vi "MyArray_client.vi"() -> ()   [LabVIEW 2010]
uses:
  src/i3-json-1.0.0-10/JSON Generation/Create Value Files/Create Value - Object.vi
  src/i3-json-1.0.0-10/JSON Generation/Add Object Parameter Files/Add Object Parameter - Numeric.vi
  src/i3-json-1.0.0-10/JSON Parsing/Get Array Value at Index Files/Get Array Value at Index - Numeric.vi
  src/i3-json-1.0.0-10/i3-json.lvlib
panel:
  out "result":dbl[](array[numeric])
  in  "n":i32=100
  out "error out":errorcluster
  in  "function name":string="linspace"
  in  "Service name":string="MyArray"
  in  "Network Manager IP Address or Hostname":string
  in  "Network Manager port":u16=1875
  in  "stop":i32=100
  in  "start":i32=10
  # "The MyArray Service\nis included with\nMSL-Network"
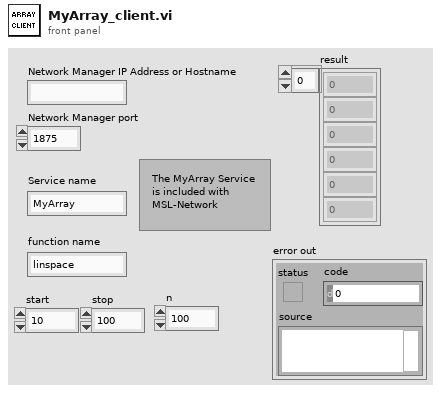
[diagram p1: front panel]
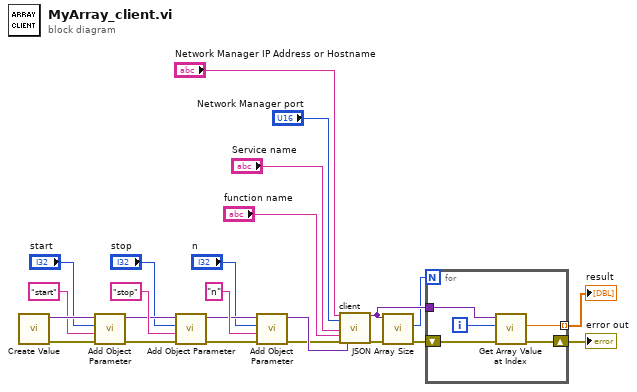
[diagram p0: block diagram]
diagram:
  n1 = call-poly "Create Value.vi"() -> ("error out"=w19:errorcluster, "JSON Tree"=w20:variant)  [unwired: 10 in]
  n2 = call-poly "Add Object Parameter.vi"("error in (no error)"=w19, "Name"="start", "Numeric"="start", "JSON Tree in (JSON Object)"=w20) -> ("error out"=w14:errorcluster, "JSON Tree out (JSON Object)"=w15:variant)  [unwired: 6 in]
  n3 = call-poly "Add Object Parameter.vi"("error in (no error)"=w14, "Name"="stop", "Numeric"="stop", "JSON Tree in (JSON Object)"=w15) -> ("error out"=w9:errorcluster, "JSON Tree out (JSON Object)"=w11:variant)  [unwired: 6 in]
  n4 = call-poly "Add Object Parameter.vi"("error in (no error)"=w9, "Name"="n", "Numeric"="n", "JSON Tree in (JSON Object)"=w11) -> ("error out"=w7:errorcluster, "JSON Tree out (JSON Object)"=w8:variant)  [unwired: 6 in]
  n5 = call "client.vi"("Network Manager IP Address or Hostname"="Network Manager IP Address or Hostname", "Network Manager port"="Network Manager port", "Service name"="Service name", "function name"="function name", "error in"=w7, "kwargs"=w8) -> ("result"=w6:variant, "error out"=w5:errorcluster)  [unwired: 12 in]
  n6 = call "JSON Array Size.vi"("error in (no error)"=w5, "JSON Tree In (JSON Array)"=w6) -> ("error out"=w3:errorcluster, "Array Size"=w2:i32)  [unwired: 7 in, 1 out]
  n7 = for {
    N: w2 -> [_]
    tunnel: w6 -> [w29]
    tunnel: [w27] -> w4 mode=indexing
    shift-right: [w25] -> w1
    shift-left: w3 -> [w26]
    i -> [w28]
    n8 = call-poly "Get Array Value at Index.vi"("error in (no error)"=w26, "Index"=w28, "JSON Tree In (JSON Array)"=w29) -> ("error out"=w25:errorcluster, "Double Value"=w27:dbl)  [unwired: 5 in, 2 out]
  }
  "error out" <- w1
  "result" <- w4
